vi "Ui.vi"() -> ()   [LabVIEW 2014, in "FPGA Module tests.lvlib"]
uses:
  FPGA Module tests.lvlib
panel:
  out "Boolean Indicator":bool
  out "FXP Indicator":dbl
  out "I32 Indicator":i32
  out "SGL Indicator":sgl
  in  "Boolean Control":bool
  in  "FXP Control":dbl
  in  "I32 Control":i32
  in  "SGL Control":sgl
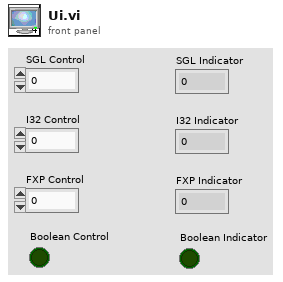
[diagram p1: front panel]
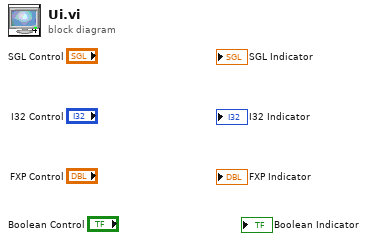
[diagram p0: block diagram]
diagram:
